vi "Write MultCol Listbox Headers.vi"(8 "error in":errorcluster, 9 "Row Headers":string[](array[string]), 10 "Column Headers":string[](array[string]), 11 "Multicolumn Listbox Ref in":refnum<vi>) -> (0 "error out":errorcluster, 3 "Multicolumn Listbox Ref out":refnum<vi>)   [LabVIEW 2020, in "G-Unicode.lvlib"]
uses:
  Unicode/Controls/String Encoding.ctl
  G-Unicode.lvlib
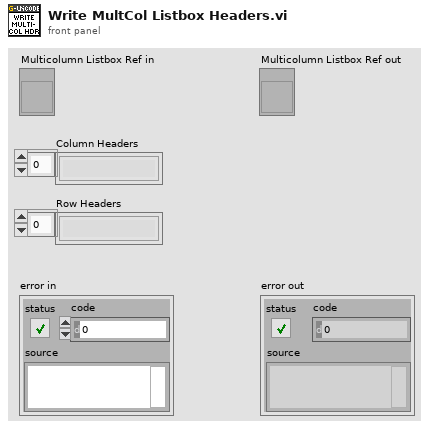
[diagram p1: front panel]
types:
  T1 = typedef "G-Unicode.lvlib/String Encoding.ctl" = enum16{"ANSI", "UTF-8", "UTF-16LE", "UTF-16BE", "Unknown"}
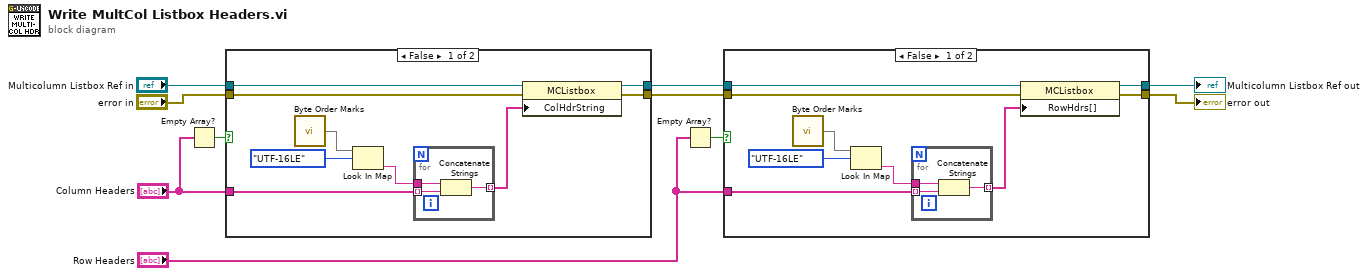
[diagram p0: block diagram]
diagram:
  n1 = Empty Array?(array="Column Headers") -> (empty?=w7:bool)
  n2 = case shown="False" w7 {
    tunnel: "error in" -> [w19 w23]
    tunnel: [w18 w23] -> w5
    tunnel: "Multicolumn Listbox Ref in" -> [w17 w24]
    tunnel: [w16 w24] -> w6
    tunnel: "Column Headers" -> [w12 _]
    frame False {
      n3 = call "Byte Order Marks.vi"() -> ("BOMs"=w15:map{T1, string})
      n4 = Look In Map(map=w15, key=String_Encoding."UTF-16LE") -> (value=w13:string)  [unwired: 1 in, 1 out]
      n5 = for {
        tunnel: w12 -> [w22] mode=indexing
        tunnel: [w21] -> w11 mode=indexing
        tunnel: w13 -> [w20]
        n6 = Concatenate Strings(w20, w22) -> (w21:string)
      }
      n7 = property class="MCListbox"(reference=w17, error in=w19, "ColHdrString"=w11) -> (reference out=w16:refnum<vi>, error out=w18:errorcluster)
    }
    frame True {
    }
  }
  n8 = Empty Array?(array="Row Headers") -> (empty?=w4:bool)
  n9 = case shown="False" w4 {
    tunnel: w5 -> [w33 w37]
    tunnel: [w32 w37] -> w1
    tunnel: w6 -> [w31 w38]
    tunnel: [w30 w38] -> w2
    tunnel: "Row Headers" -> [w26 _]
    frame False {
      n10 = call "Byte Order Marks.vi"() -> ("BOMs"=w29:map{T1, string})
      n11 = Look In Map(map=w29, key=String_Encoding."UTF-16LE") -> (value=w27:string)  [unwired: 1 in, 1 out]
      n12 = for {
        tunnel: w26 -> [w36] mode=indexing
        tunnel: [w35] -> w25 mode=indexing
        tunnel: w27 -> [w34]
        n13 = Concatenate Strings(w34, w36) -> (w35:string)
      }
      n14 = property class="MCListbox"(reference=w31, error in=w33, "RowHdrs[]"=w25) -> (reference out=w30:refnum<vi>, error out=w32:errorcluster)
    }
    frame True {
    }
  }
  "error out" <- w1
  "Multicolumn Listbox Ref out" <- w2
